vi "Trigger flanco (SubVI).vi"(8 "Slope":u16(ring) items=["Fall", "Rise"], 9 "Acoplamiento":u16(ring) items=["AC", "DC", "Sin altas frecuencias DC", "Sin bajas frecuencias AC", "Baja sensibilidad DC"], 10 "Canal":u16(ring) items=["Canal 1", "Canal 2"], 11 "String de Entrada":string) -> (2 "String de Salida":string, 3 "String de tipo":string)   [LabVIEW 2019]
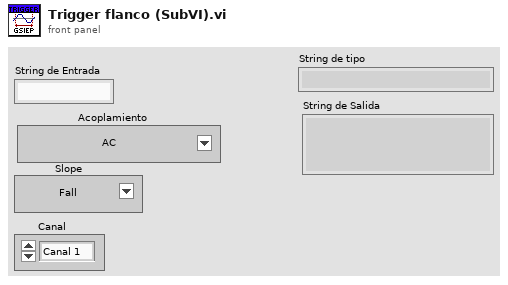
[diagram p1: front panel]
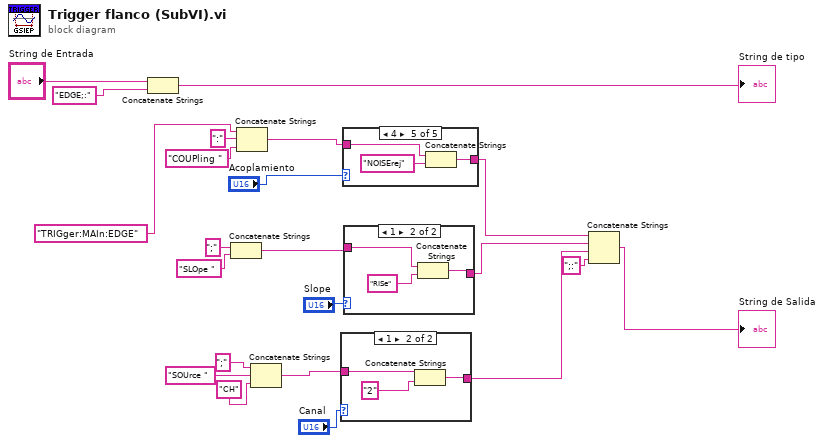
[diagram p0: block diagram]
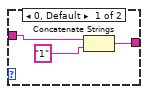
[diagram p2: hidden frame]
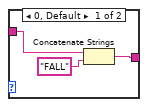
[diagram p3: hidden frame]
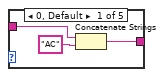
[diagram p4: hidden frame]
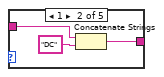
[diagram p5: hidden frame]
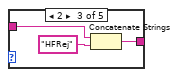
[diagram p6: hidden frame]
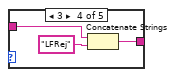
[diagram p7: hidden frame]
diagram:
  n1 = Concatenate Strings("String de Entrada", "EDGE;:") -> (→"String de tipo":string)
  n2 = Concatenate Strings(";", "SLOpe ") -> (w11:string)
  n3 = Concatenate Strings("TRIGger:MAIn:EDGE", ":", "COUPling ") -> (w5:string)
  n4 = Concatenate Strings(";", "SOUrce ", "CH") -> (w13:string)
  n5 = case shown="1" "Canal" {
    tunnel: w13 -> [w24 w27]
    tunnel: [w23 w26] -> w20
    frame 0, Default {
      n6 = Concatenate Strings(w24, "1") -> (w23:string)
    }
    frame 1 {
      n7 = Concatenate Strings(w27, "2") -> (w26:string)
    }
  }
  n8 = case shown="4" "Acoplamiento" {
    tunnel: w5 -> [w30 w33 w36 w39 w42]
    tunnel: [w29 w32 w35 w38 w41] -> w18
    frame 0, Default {
      n9 = Concatenate Strings(w30, "AC") -> (w29:string)
    }
    frame 1 {
      n10 = Concatenate Strings(w33, "DC") -> (w32:string)
    }
    frame 2 {
      n11 = Concatenate Strings(w36, "HFRej") -> (w35:string)
    }
    frame 3 {
      n12 = Concatenate Strings(w39, "LFRej") -> (w38:string)
    }
    frame 4 {
      n13 = Concatenate Strings(w42, "NOISErej") -> (w41:string)
    }
  }
  n14 = case shown="1" "Slope" {
    tunnel: w11 -> [w45 w48]
    tunnel: [w44 w47] -> w19
    frame 0, Default {
      n15 = Concatenate Strings(w45, "FALL") -> (w44:string)
    }
    frame 1 {
      n16 = Concatenate Strings(w48, "RISe") -> (w47:string)
    }
  }
  n17 = Concatenate Strings(w18, w19, w20, ";:") -> (→"String de Salida":string)
